vi "Find Circles.vi"() -> ()   [LabVIEW 2020]
uses:
  feature_detection/Hough Circle Result.ctl
  common/Image Point (Float).ctl
  image/Image Read Size.ctl
  image/Kernel Block Size.ctl
  feature_detection/Hough Circle Parameters.ctl
  feature_detection/Hough Circle Modes.ctl
  image/Canny Aperture Size.ctl
  image/ARGB Colour.ctl
  image/New Image (ARGB).vi
  image/Read Image File (ARGB).vi
  image/Draw Image to Picture (ARGB).vi
  image/Blur (Gaussian Greyscale).vi
  image/Threshold (Binary).vi
  image/Draw Image to Picture (Greyscale).vi
  image/Draw Circle (ARGB).vi
  image/New Image (ARGB).vi/3321fa97-f432-4e1e-8db9-a0df79aed21b.vi
  image/ARGB Colour to U32 Pixel Value.vi
  image/Read Image File (ARGB).vi/2358f293-6357-4b7a-bec3-c4e4d03be6e5.vi
  image/Draw Image to Picture (ARGB).vi/8cd07b1b-062e-4fe4-9e87-2eb3dc89fe0e.vi
  image/New Image (Greyscale).vi/6598b9e0-8a08-46f5-91fd-ca1b87217137.vi
  image/ARGBExtractChannel.vi
  image/Blur (Gaussian Greyscale).vi/68bb216c-d3e3-4366-946f-f5b7f5c74ae7.vi
  image/ThresholdCore.vi
  image/Draw Image to Picture (Greyscale).vi/9ae995ca-ccda-485c-89ac-02736fde3e8e.vi
  image/Draw Circle (ARGB).vi/8336a1cf-e433-4bea-8080-376bdb783d4e.vi
  common/Module Path.vi
  <vilib>/Utility/error.llb/Error Cluster From Error Code.vi
  image/image.lvlib
  feature_detection/feature_detection.lvlib
  common/common.lvlib
panel:
  in  "Image to Binary Mode":enum16{"Threshold", "Canny Edges"}(ring)
  out "Results":T1[](array[typedef])
  out "Input":picture
  out "Blur & Binary":picture
  out "Draw Overlay":picture
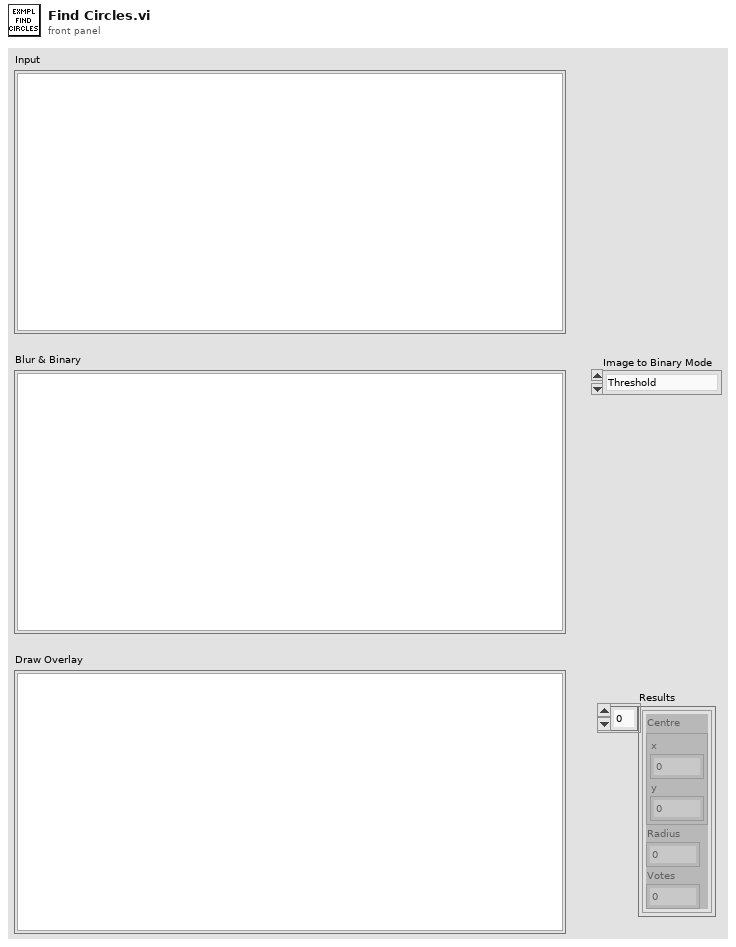
[diagram p1: front panel]
types:
  T1 = typedef "feature_detection.lvlib/Hough Circle Result.ctl" = cluster{"Centre":T2, "Radius":dbl, "Votes":dbl}
  T2 = typedef "common.lvlib/Image Point (Float).ctl" = cluster{"x":dbl, "y":dbl}
  T3 = typedef "feature_detection.lvlib/Hough Circle Modes.ctl" = enum16{"GRADIENT", "GRADIENT_ALT"}
  T4 = typedef "feature_detection.lvlib/Hough Circle Parameters.ctl" = cluster{"Param1":dbl, "Param2":dbl, "Minimum Radius":i32, "Maximum Radius":i32}
  T5 = typedef "image.lvlib/Kernel Block Size.ctl" = enum16{"3", "5", "7", "9", "11", "13", "15", "17", "19", "21", "23", "25", "27", "29", "31", "33", "35", "37", "39", "41", "43", "45", "47", "49", "51", "53", "55", "57", "59", "61", "63", "65", "67", "69", "71", "73", "75", "77", "79", "81", "83", "85", "87", "89", "91", "93", "95", "97", "99", "101", "103", "105", "107", "109", "111", "113", "115", "117", "119", "121", "123", "125", "127", "129", "131", "133", "135", "137", "139", "141", "143", "145", "147", "149", "151", "153", "155", "157", "159", "161", "163", "165", "167", "169", "171", "173", "175", "177", "179", "181", "183", "185", "187", "189", "191", "193", "195", "197", "199", "201", "203", "205", "207", "209", "211", "213", "215", "217", "219", "221", "223", "225", "227", "229", "231", "233", "235", "237", "239", "241", "243", "245", "247", "249", "251", "253", "255", "257", "259", "261", "263", "265", "267", "269", "271", "273", "275", "277", "279", "281", "283", "285", "287", "289", "291", "293", "295", "297", "299", "301", "303", "305", "307", "309", "311", "313", "315", "317", "319", "321", "323", "325", "327", "329", "331", "333", "335", "337", "339", "341", "343", "345", "347", "349", "351", "353", "355", "357"}
  T6 = typedef "image.lvlib/Image Read Size.ctl" = enum8{"FULL_SIZE", "REDUCED_2", "REDUCED_4", "REDUCED_8"}
  T7 = typedef "image.lvlib/ARGB Image.ctl" = refnum<data-value>
  T8 = typedef "image.lvlib/Greyscale Image.ctl" = refnum<data-value>
  T9 = typedef "image.lvlib/Canny Aperture Size.ctl" = enum16{"3", "5", "7"}
  T10 = typedef "image.lvlib/ARGB Colour.ctl" = cluster{"Alpha":u8, "RGB":u32}
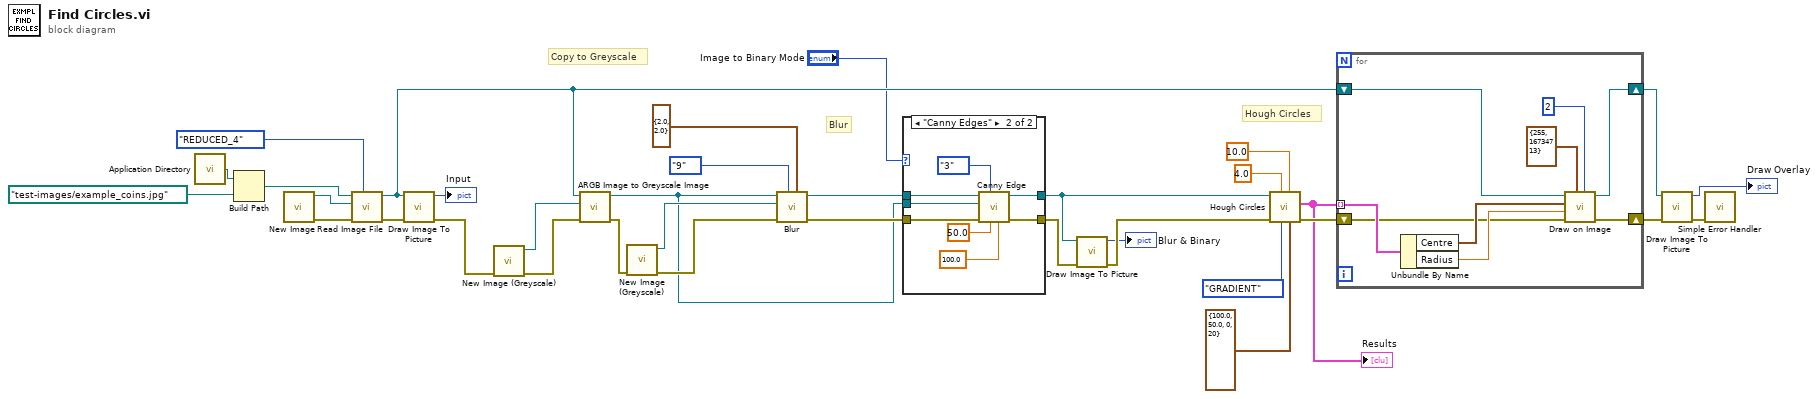
[diagram p0: block diagram]
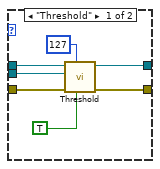
[diagram p2: hidden frame]
diagram:
  # "Hough Circles"
  # "Blur"
  # "Copy to Greyscale"
  n1 = call <vilib>:"Application Directory.vi"() -> ("Application Directory"=w26:path)
  n2 = Build Path(base path=w26, name or relative path=path "test-images/example_coins.jpg" ("Path")) -> (appended path=w35:path)
  n3 = call-poly "New Image.vi"() -> ("error out"=w33:errorcluster, "New ARGB Image"=w34:T7)  [unwired: 10 in]
  n4 = call-poly "Read Image File.vi"("Image Read Size (Default: FULL_SIZE)"=Image_Read_Size."REDUCED_4", "error in (no error)"=w33, "ARGB Image Destination"=w34, "Filepath"=w35) -> ("error out"=w20:errorcluster, "ARGB Image Destination (duplicate)"=w21:T7)  [unwired: 6 in]
  n5 = call-poly "Draw Image To Picture.vi"("error in (no error)"=w20, "ARGB Image Source"=w21) -> ("error out"=w19:errorcluster, "Picture"=→"Input":picture)  [unwired: 8 in]
  n6 = call "New Image (Greyscale).vi"("error in (no error)"=w19) -> ("error out"=w25:errorcluster, "New Greyscale Image"=w24:T8)  [unwired: 9 in]
  n7 = call "ARGB Image to Greyscale Image.vi"("error in (no error)"=w25, "Greyscale Image Destination"=w24, "ARGB Image Source"=w21) -> ("error out"=w13:errorcluster, "Greyscale Image Destination (Duplicate)"=w2:T8)  [unwired: 7 in]
  n8 = call "New Image (Greyscale).vi"("error in (no error)"=w13) -> ("error out"=w12:errorcluster, "New Greyscale Image"=w10:T8)  [unwired: 9 in]
  n9 = call-poly "Blur.vi"("Sigma"=T2 {"x"=2.0, "y"=2.0}, "Kernel Block Size"=Kernel_Block_Size."9", "error in (no error)"=w12, "Gaussian Blur Result"=w10, "Greyscale Image-Source"=w2) -> ("error out"=w3:errorcluster, "Gaussian Blur Result (duplicate)"=w11:T8)  [unwired: 5 in]
  n10 = case shown="\"Canny Edges\"" "Image to Binary Mode" {
    tunnel: [w37 w50] -> w18
    tunnel: [w38 w49] -> w16
    tunnel: w11 -> [w40 w48]
    tunnel: w3 -> [w41 w47]
    tunnel: w2 -> [w39 w46]
    frame "Threshold" {
      n11 = call-poly "Threshold.vi"("Invert? (Default: False)"=TRUE, "Threshold"=u8 127, "error in (no error)"=w41, "Threshold Result"=w39, "Greyscale Image-Source"=w40) -> ("error out"=w37:errorcluster, "Threshold Result (duplicate)"=w38:T8)  [unwired: 5 in]
    }
    frame "Canny Edges" {
      n12 = call "Canny Edge.vi"("Threshold 2"=100.0, "Threshold 1"=50.0, "Aperture Size"=Canny_Aperture_Size."3", "error in (no error)"=w47, "Canny Edge Result"=w46, "Greyscale Image-Source"=w48) -> ("error out"=w50:errorcluster, "Canny Edge (duplicate)"=w49:T8)  [unwired: 4 in]
    }
  }
  n13 = call-poly "Draw Image To Picture.vi"("error in (no error)"=w18, "Greyscale Image Source"=w16) -> ("error out"=w17:errorcluster, "Picture"=→"Blur & Binary":picture)  [unwired: 8 in]
  n14 = call "Hough Circles.vi"("Hough Circle Parameters (Default: OpenCV Defaults)"=T4 {"Param1"=100.0, "Param2"=50.0, "Minimum Radius"=0, "Maximum Radius"=20}, "Minimum Distance"=10.0, "Hough Circle Modes (Default: GRADIENT)"=Hough_Circle_Modes."GRADIENT", "DP"=4.0, "error in (no error)"=w17, "Greyscale Image"=w16) -> ("error out"=w29:errorcluster, "Results"=w28:T1[])  [unwired: 3 in, 1 out]
  "Results" <- w28
  n15 = for {
    shift-right: [w59] -> w30
    shift-left: w29 -> [w53]
    tunnel: w28 -> [w58] mode=indexing
    shift-right: [w57] -> w23
    shift-left: w21 -> [w54]
    n16 = Unbundle By Name(w58) -> ("Centre"=w56:T2, "Radius"=w55:dbl)
    n17 = call-poly "Draw on Image.vi"("Thickness (Default: 1)"=2, "ARGB Colour"=T10 {"Alpha"=255, "RGB"=16734713}, "error in (no error)"=w53, "Radius"=w55, "Centre"=w56, "ARGB Image"=w54) -> ("error out"=w59:errorcluster, "ARGB Image (Duplicate)"=w57:T7)  [unwired: 4 in]
  }
  n18 = call-poly "Draw Image To Picture.vi"("error in (no error)"=w30, "ARGB Image Source"=w23) -> ("error out"=w22:errorcluster, "Picture"=→"Draw Overlay":picture)  [unwired: 8 in]
  n19 = call <vilib>:"Simple Error Handler.vi"("error in (no error)"=w22) -> ()  [unwired: 4 in, 5 out]
